vi "Traverse Ctrl.vi"(8 "error in":errorcluster, 10 "VISA resource name":refnum<visa-resource-name>, 11 "Water Tunnel Results in":refnum<class "Water Tunnel Results.lvclass">) -> (0 "error out":errorcluster, 2 "VISA resource name out":refnum<visa-resource-name>, 3 "Water Tunnel Results out":refnum<class "Water Tunnel Results.lvclass">)   [LabVIEW 2019, in "Results.lvlib" / "Water Tunnel Results.lvclass"]
uses:
  Water Tunnel Results.lvclass
  Water Tunnel Results.lvclass/Water Tunnel Results.ctl
panel:
  out "Wing aligned?":bool
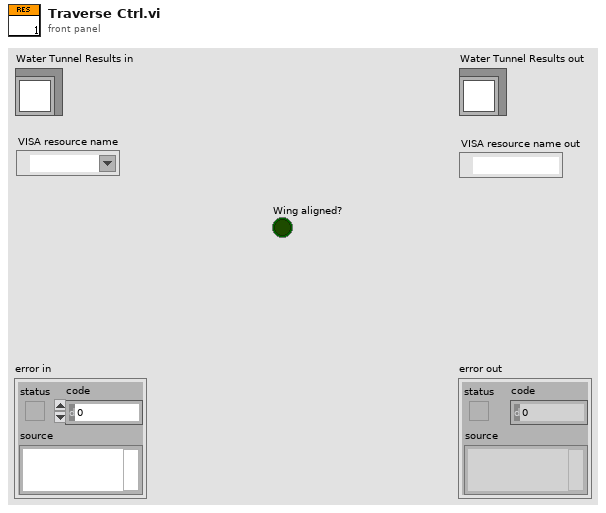
[diagram p1: front panel]
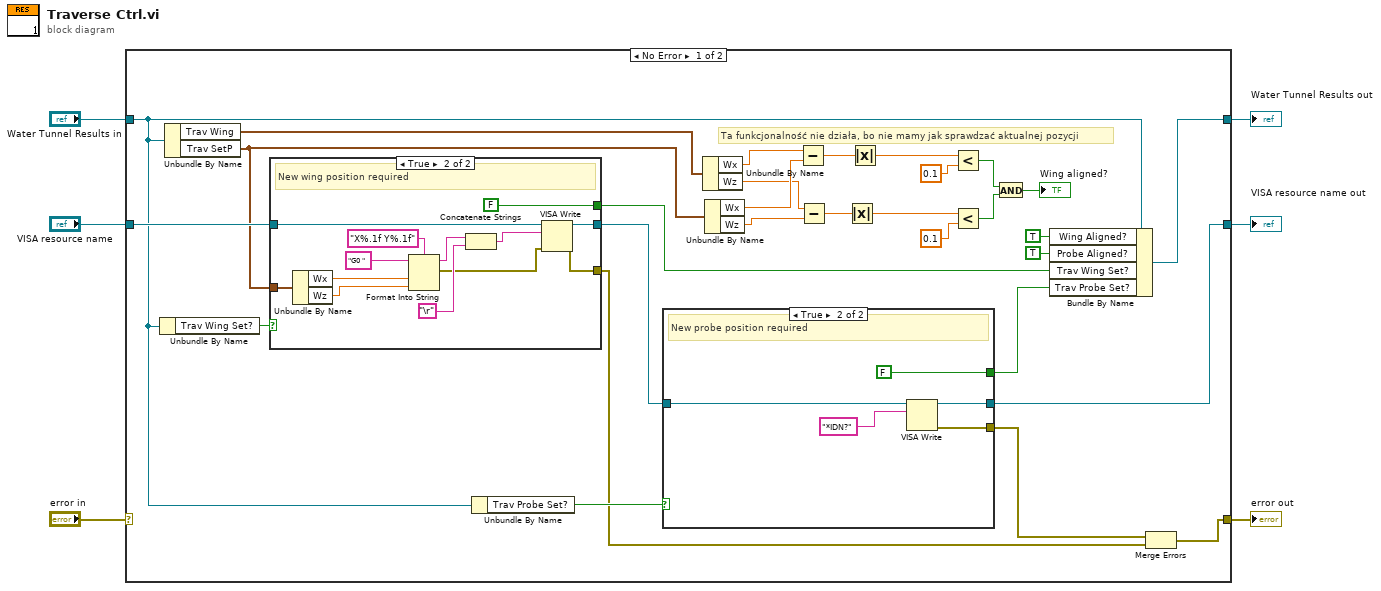
[diagram p0: block diagram]
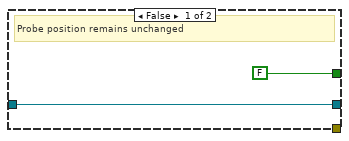
[diagram p2: hidden frame]
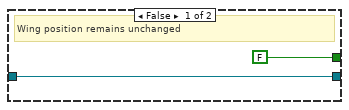
[diagram p3: hidden frame]
diagram:
  n1 = case shown="No Error" "error in" {
    selector: "error in" -> [_ w60]
    tunnel: [w27 w60] -> w5
    tunnel: [w35 w59] -> w3
    tunnel: "Water Tunnel Results in" -> [w7 w59]
    tunnel: "VISA resource name" -> [w33 w58]
    tunnel: [w30 w58] -> w1
    frame No Error {
      # "Ta funkcjonalność nie działa, bo nie mamy jak sprawdzać aktualnej pozycji"
      n2 = Unbundle By Name(w7) -> ("Trav Wing Set?"=w34:bool)
      n3 = Unbundle By Name(w7) -> ("Trav Wing"=w24:cluster{"Wx":dbl, "Wz":dbl, "Wa":dbl}, "Trav SetP"=w23:cluster{"Wx":dbl, "Wz":dbl, "Wa":dbl, "Pz":dbl})
      n4 = case shown="True" w34 {
        tunnel: w33 -> [w43 w57]
        tunnel: [FALSE FALSE] -> w26
        tunnel: [w43 w55] -> w31
        tunnel: [_ w54] -> w29
        tunnel: w23 -> [_ w53]
        frame False {
          # "Wing position remains unchanged"
        }
        frame True {
          # "New wing position required"
          n5 = Unbundle By Name(w53) -> ("Wx"=w50:dbl, "Wz"=w49:dbl)
          n6 = Format Into String(format string="X%.1f Y%.1f", initial string="G0 ", w50, w49) -> (resulting string=w48:string, error out=w45:errorcluster)  [unwired: 1 in]
          n7 = Concatenate Strings(w48, "\r") -> (w46:string)
          n8 = VISA Write(VISA resource name=w57, write buffer=w46, error in (no error)=w45) -> (VISA resource name out=w55:refnum<visa-resource-name>, error out=w54:errorcluster)  [unwired: 1 out]
        }
      }
      n9 = Unbundle By Name(w7) -> ("Trav Probe Set?"=w32:bool)
      n10 = case shown="True" w32 {
        tunnel: w31 -> [w36 w42]
        tunnel: [FALSE FALSE] -> w25
        tunnel: [w36 w39] -> w30
        tunnel: [_ w38] -> w28
        frame False {
          # "Probe position remains unchanged"
        }
        frame True {
          # "New probe position required"
          n11 = VISA Write(VISA resource name=w42, write buffer="*IDN?") -> (VISA resource name out=w39:refnum<visa-resource-name>, error out=w38:errorcluster)  [unwired: 1 in, 1 out]
        }
      }
      n12 = Unbundle By Name(w24) -> ("Wx"=w22:dbl, "Wz"=w20:dbl)
      n13 = Unbundle By Name(w23) -> ("Wx"=w21:dbl, "Wz"=w19:dbl)
      n14 = Subtract(x=w22, y=w21) -> (x-y=w18:dbl)
      n15 = Subtract(x=w20, y=w19) -> (x-y=w15:dbl)
      n16 = Absolute Value(x=w15) -> (abs(x)=w10:dbl)
      n17 = Absolute Value(x=w18) -> (abs(x)=w11:dbl)
      n18 = Less?(x=w11, y=0.1) -> (x < y?=w14:bool)
      n19 = Less?(x=w10, y=0.1) -> (x < y?=w13:bool)
      n20 = And(x=w14, y=w13) -> (x .and. y?=→"Wing aligned?":bool)
      n21 = Bundle By Name(cluster=w7, "Wing Aligned?"=TRUE, "Probe Aligned?"=TRUE, "Trav Wing Set?"=w26, "Trav Probe Set?"=w25) -> (w35:refnum<class "Water Tunnel Results.lvclass">)
      n22 = Merge Errors(w28, w29) -> (w27:errorcluster)
    }
    frame Error {
    }
  }
  "error out" <- w5
  "Water Tunnel Results out" <- w3
  "VISA resource name out" <- w1
